vi "more_10_flag.vi"(1 "input":T1) -> (0 "flag":bool)   [LabVIEW 2013]
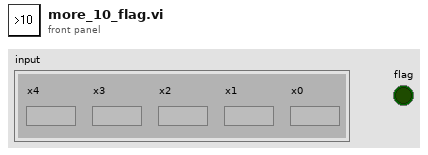
[diagram p1: front panel]
types:
  T1 = cluster{"x4":bool, "x3":bool, "x2":bool, "x1":bool, "x0":bool}
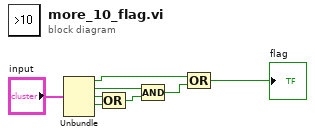
[diagram p0: block diagram]
diagram:
  n1 = Unbundle("input") -> ("x4"=w3:bool, "x3"=w7:bool, "x2"=w6:bool, "x1"=w5:bool)  [unwired: 1 out]
  n2 = Compound Arithmetic op=OR(w6, w5) -> (w4:bool)
  n3 = Compound Arithmetic op=AND(w7, w4) -> (w2:bool)
  n4 = Compound Arithmetic op=OR(w3, w2) -> (→"flag":bool)
